vi "SetToDefault.vi"(8 "error in (no error)":errorcluster, 11 "Menu in":refnum<class "MGI_Menu.lvclass">) -> (0 "error out":errorcluster, 3 "Menu out":refnum<class "MGI_Menu.lvclass">)   [LabVIEW 2016, in "MGI_Menu.lvclass"]
doc: "Searches the menu for any item with \"Clicked by Default\" set to true and then fakes a click on this item. This is useful for initializeing radio selections or checkmark selections to default values.\n\nMenuItem Clicked Events will be generates for these default clicks. If you want to process these events, make sure this VI is run after the Register for User Events node on the MenuItem Clicked Event.\n\nAuthored by Derek E. Trepanier\nsupport@mooregoodideas.com\nwww.mooregoodideas.com\n\nCopyright (c) 2012, Moore Good Ideas, Inc.\n\nAll rights reserved.\n\nRedistribution and use in source and binary forms, with or without modification, are permitted provided that the following conditions are met:\n\n * Redistributions of source code must retain the above copyright notice, this list of conditions and the following disclaimer.\n * Redistributions in binary form must reproduce the above copyright notice, this list of conditions and the following disclaimer in the documentation and/or other materials provided with the distribution.\n * Neither the name of Moore Good Ideas, Inc. nor the names of its contributors may be used to endorse or promote products derived from this software without specific prior written permission.\n\nTHIS SOFTWARE IS PROVIDED BY THE COPYRIGHT HOLDERS AND CONTRIBUTORS \"AS IS\" AND ANY EXPRESS OR IMPLIED WARRANTIES, INCLUDING, BUT NOT LIMITED TO, THE IMPLIED WARRANTIES OF MERCHANTABILITY AND FITNESS FOR A PARTICULAR PURPOSE ARE DISCLAIMED. IN NO EVENT SHALL THE COPYRIGHT OWNER OR CONTRIBUTORS BE LIABLE FOR ANY DIRECT, INDIRECT, INCIDENTAL, SPECIAL, EXEMPLARY, OR CONSEQUENTIAL DAMAGES (INCLUDING, BUT NOT LIMITED TO, PROCUREMENT OF SUBSTITUTE GOODS OR SERVICES; LOSS OF USE, DATA, OR PROFITS; OR BUSINESS INTERRUPTION) HOWEVER CAUSED AND ON ANY THEORY OF LIABILITY, WHETHER IN CONTRACT, STRICT LIABILITY, OR TORT (INCLUDING NEGLIGENCE OR OTHERWISE) ARISING IN ANY WAY OUT OF THE USE OF THIS SOFTWARE, EVEN IF ADVISED OF THE POSSIBILITY OF SUCH DAMAGE."
uses:
  <userlib>/_MGI/Menu Building/MenuTypes/MGI_Menu.lvclass
  <userlib>/_MGI/Menu Building/MenuTypes/MGI_Menu.lvclass/MGI_Menu.ctl
  <userlib>/_MGI/Menu Building/MenuItem/MGI_MenuItem.lvclass
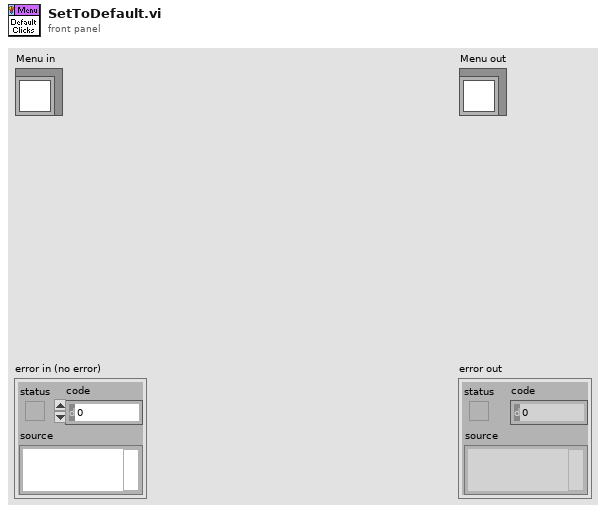
[diagram p1: front panel]
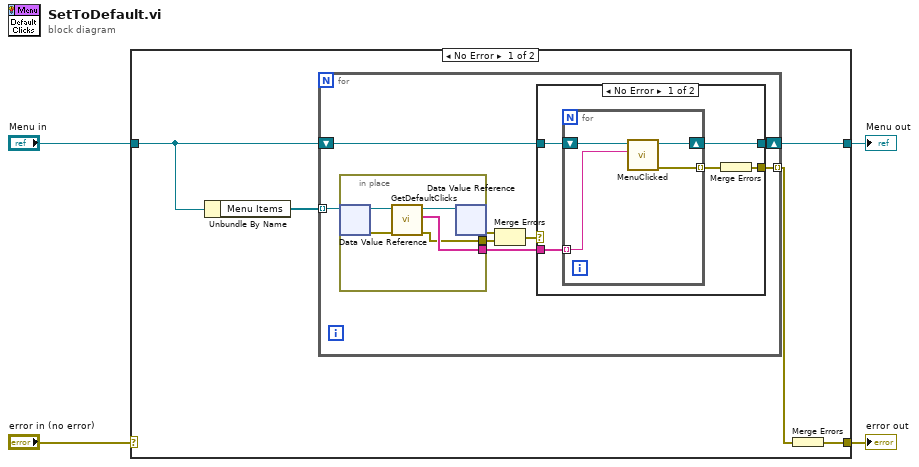
[diagram p0: block diagram]
diagram:
  n1 = case shown="No Error" "error in (no error)" {
    selector: "error in (no error)" -> [_ w34]
    tunnel: [w5 w34] -> w3
    tunnel: [w7 w33] -> w1
    tunnel: "Menu in" -> [w8 w33]
    frame No Error {
      n2 = Unbundle By Name(w8) -> ("Menu Items"=w9:refnum<data-value>[])
      n3 = for {
        tunnel: w9 -> [w14] mode=indexing
        shift-right: [w16] -> w7
        shift-left: w8 -> [w17]
        tunnel: [w15] -> w6 mode=indexing
        n4 = in-place {
          in-place-border: [w20] -> w13
          in-place-border: [w18] -> w10
          n5 = in-place-dvr #1(w14) -> (w22:refnum<class "MGI_MenuItem.lvclass">, w19:errorcluster)
          n6 = call <userlib>:"GetDefaultClicks.vi"("error in (no error)"=w19, "MGI_MenuItem in"=w22) -> ("error out"=w18:errorcluster, "Default Click Tags"=w20:string[], "MGI_MenuItem out"=w21:refnum<class "MGI_MenuItem.lvclass">)  [unwired: 7 in]
          n7 = in-place-dvr #1(w21) -> (w12:errorcluster)  [unwired: 1 out]
        }
        n8 = Merge Errors(w12, w10) -> (w11:errorcluster)
        n9 = case shown="No Error" w11 {
          tunnel: w17 -> [w27 w32]
          tunnel: [w26 w32] -> w16
          tunnel: [w24 _] -> w15
          tunnel: w13 -> [w23 _]
          frame No Error {
            n10 = for {
              shift-right: [w30] -> w26
              shift-left: w27 -> [w31]
              tunnel: [w29] -> w25 mode=indexing
              tunnel: w23 -> [w28] mode=indexing
              n11 = call-dynamic "MenuClicked.vi"("Full Tag"=w28, "Menu in"=w31) -> ("error out"=w29:errorcluster, "Menu out"=w30:refnum<class "MGI_Menu.lvclass">)  [unwired: 8 in]
            }
            n12 = Merge Errors(w25) -> (w24:errorcluster)
          }
          frame Error {
          }
        }
      }
      n13 = Merge Errors(w6) -> (w5:errorcluster)
    }
    frame Error {
    }
  }
  "error out" <- w3
  "Menu out" <- w1
